vi "Query Operational Condition Register.vi"(8 "error in":errorcluster, 10 "Status in":T1, 11 "6032A in":refnum<class "6032A.lvclass">) -> (0 "error out":errorcluster, 2 "Status out":T1, 3 "6032A out":refnum<class "6032A.lvclass">)   [LabVIEW 2019, in "6032A.lvlib" / "6032A.lvclass"]
uses:
  Library/6032A.lvclass
  builds/Instruments/PowerSupply.lvlibp/Custom Controls/Status_Flags.ctl
  Library/6032A.lvclass/6032A.ctl
  builds/Instruments/PowerSupply.lvlibp/Library/PowerSupply.lvclass
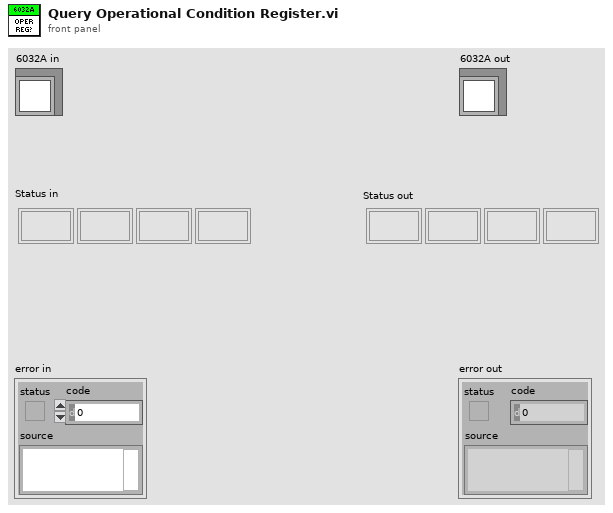
[diagram p1: front panel]
types:
  T1 = typedef "PowerSupply.lvlibp/PowerSupply.lvclass/Status_Flags.ctl" = cluster{"Interlock":bool, "OVP":bool, "OCP":bool, "Output":bool}
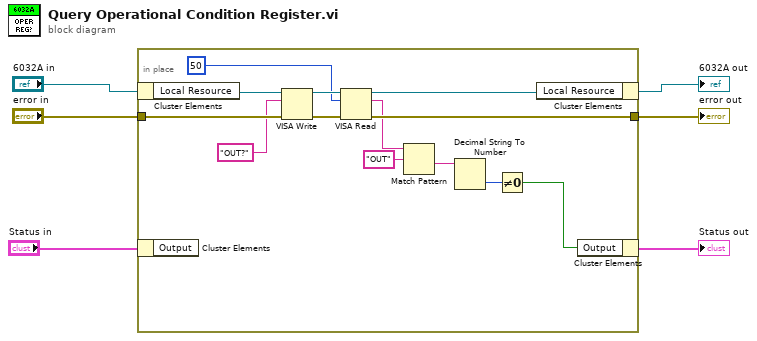
[diagram p0: block diagram]
diagram:
  n1 = in-place {
    in-place-border: [w15] -> w4
    in-place-border: "error in" -> [w14]
    n2 = in-place-cluster #1("6032A in") -> ("Local Resource"=w19:refnum<visa-resource-name>)
    n3 = in-place-cluster #2("Status in") -> ()  [unwired: 1 out]
    n4 = VISA Write(VISA resource name=w19, write buffer="OUT?", error in (no error)=w14) -> (VISA resource name out=w18:refnum<visa-resource-name>, error out=w16:errorcluster)  [unwired: 1 out]
    n5 = VISA Read(VISA resource name=w18, byte count=u32 50, error in (no error)=w16) -> (VISA resource name out=w17:refnum<visa-resource-name>, read buffer=w11:string, error out=w15:errorcluster)  [unwired: 1 out]
    n6 = Match Pattern(string=w11, regular expression="OUT") -> (after substring=w9:string)  [unwired: 1 in, 3 out]
    n7 = Decimal String To Number(string=w9) -> (number=w8:i32)  [unwired: 2 in, 1 out]
    n8 = Not Equal To 0?(x=w8) -> (x != 0?=w7:bool)
    n9 = in-place-cluster #1("Local Resource"=w17) -> (→"6032A out":refnum<class "6032A.lvclass">)
    n10 = in-place-cluster #2("Output"=w7) -> (→"Status out":T1)
  }
  "error out" <- w4
